vi "bpsk.vi"() -> ()   [LabVIEW 2016]
panel:
  out "BPSK Graph":dynamicdata(graph)
  out "Square":dynamicdata(graph)
  out "Sine":dynamicdata(graph)
  in  "SQ Freq 2":dbl(slide)=10.1 caption="Frequency" scale=0.0..50.0
  in  "Sq AMP\n 2":dbl(slide)=1.0 caption="Amplitude" scale=0.0..10.0
  in  "Sine Freq":dbl(slide)=10.1 caption="Frequency" scale=0.0..500.0
  in  "Sine AMP":dbl(slide)=1.0 caption="Amplitude" scale=0.0..10.0
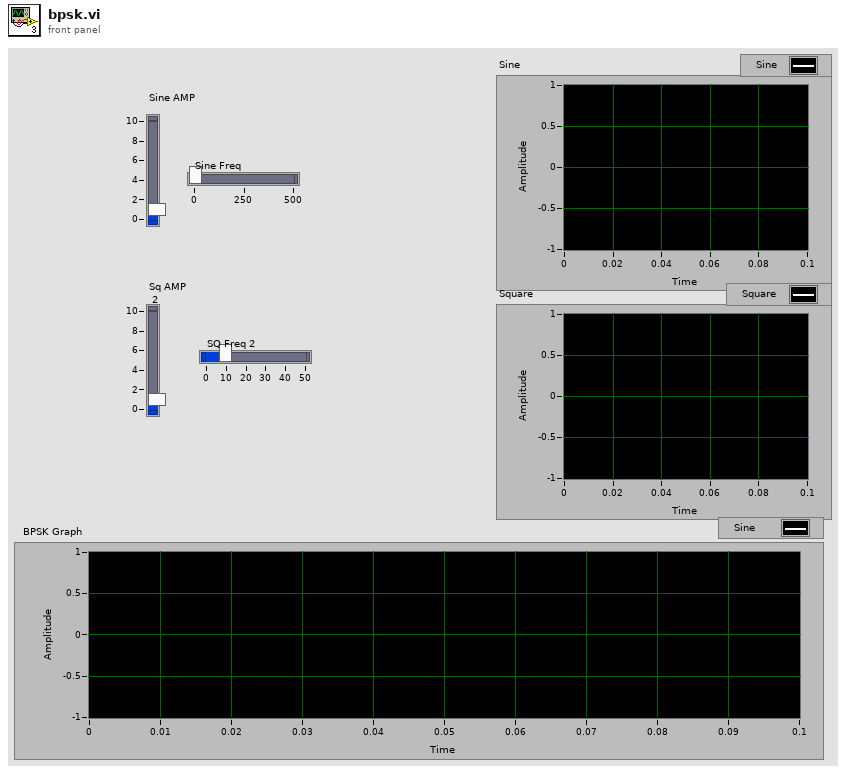
[diagram p1: front panel]
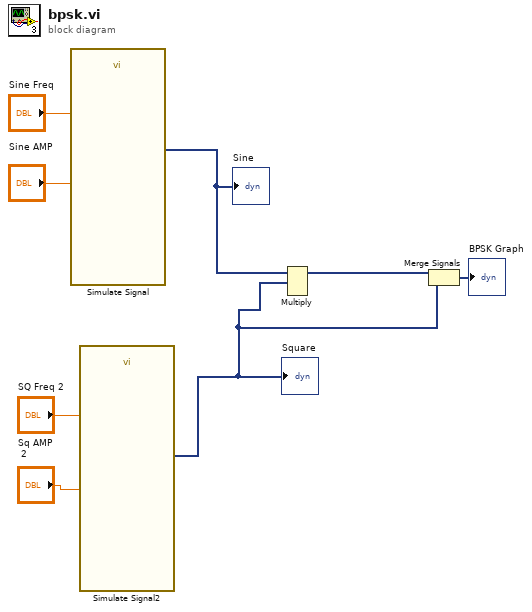
[diagram p0: block diagram]
diagram:
  n1 = call "Simulate Signal"("Frequency"="Sine Freq", "Amplitude"="Sine AMP") -> ("Sine"=w4:dynamicdata)  [unwired: 12 in, 1 out]
  "Sine" <- w4
  n2 = call "Simulate Signal2"("Frequency"="SQ Freq 2", "Amplitude"="Sq AMP\n 2") -> ("Square"=w2:dynamicdata)  [unwired: 12 in, 1 out]
  "Square" <- w2
  n3 = Multiply(1:w2, 2:w4) -> (0:w3:dynamicdata)  [unwired: 1 in, 1 out]
  n4 = Merge Signals(w3, w2) -> (→"BPSK Graph":dynamicdata)
